vi "Introduce.vi"(8 "Error In":errorcluster, 11 "BattleDroid in":refnum<class "BattleDroid.lvclass">) -> (0 "Error Out":errorcluster, 3 "BattleDroid out":refnum<class "BattleDroid.lvclass">)   [LabVIEW 2021, in "BattleDroid.lvclass"]
doc: "Show ID of droid in prompt message for user. Comments in Polish."
uses:
  BattleDroid.lvclass
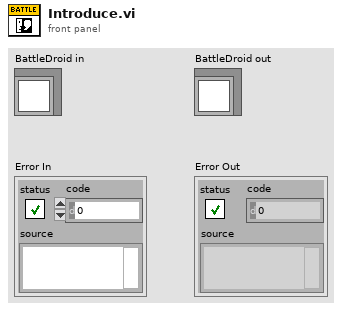
[diagram p1: front panel]
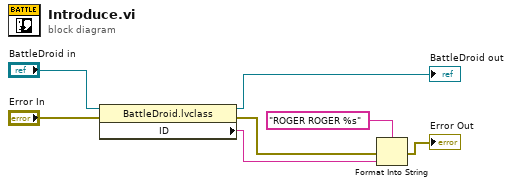
[diagram p0: block diagram]
diagram:
  n1 = property class="BattleDroid.lvclass"(reference="BattleDroid in", error in="Error In") -> (reference out=→"BattleDroid out":refnum<class "BattleDroid.lvclass">, error out=w2:errorcluster, "ID"=w3:string)
  n2 = Format Into String(format string="ROGER ROGER %s", error in=w2, w3) -> (error out=→"Error Out":errorcluster)  [unwired: 1 in, 1 out]
